vi "example.vi"() -> ()   [LabVIEW 2017, in "libfreenect.lvlib"]
uses:
  libfreenect.lvlib
  <vilib>/Analysis/coordinate.llb/2D Cartesian Coordinate Rotation (Array).vi
  <vilib>/gmath/statdist.llb/Normal PDF.vi
  <vilib>/Analysis/NI_AALPro.lvlib
  <vilib>/gmath/NI_Gmath.lvlib
panel:
  out "KINECT DATA":cluster{dbl[], dbl[]}[](graph)
  in  "Till Angle":dbl(slide) scale=-31.0..31.0 scale format="%#_5g"
  out "Heading":dbl(knob) scale=-180.0..180.0
  in  "Start":bool
  out "Command String":string
  out "Roll":dbl(knob) scale=-180.0..180.0
  out "Pitch":dbl(slide) scale=-90.0..90.0
  in  "Stop Continuous":bool
  out "Error Output":errorcluster
  in  "Serial Port":refnum<visa-resource-name>="COM1"
  in  "Baud Rate":u32=115200
  in  "std":dbl=1.0
  in  "x":dbl=50.0
  in  "y":dbl=50.0
  in  "x":dbl
  in  "y1":dbl
  out "Occupancy Grid Map":dbl[][](graph)
  in  "x1":dbl
  out "z":dbl
  out "y":dbl
  out "x":dbl
  in  "error in (no error)":errorcluster
  out "H-A":dbl
  out "W-A":dbl
  out "Height":dbl
  out "Width":dbl
  out "Depth Image":T1(plugin-control)
  out "RGB Image":T1(plugin-control)
  in  "stop":bool
  out "Range":dbl
  # "KINECT CONTROL BUTTONS"
  # "Pixel Coordinate"
  # "Map Coordinates"
  # "DATA IMAGE"
  # "IMU CONTROL BUTTONS"
  # "IMU DATA"
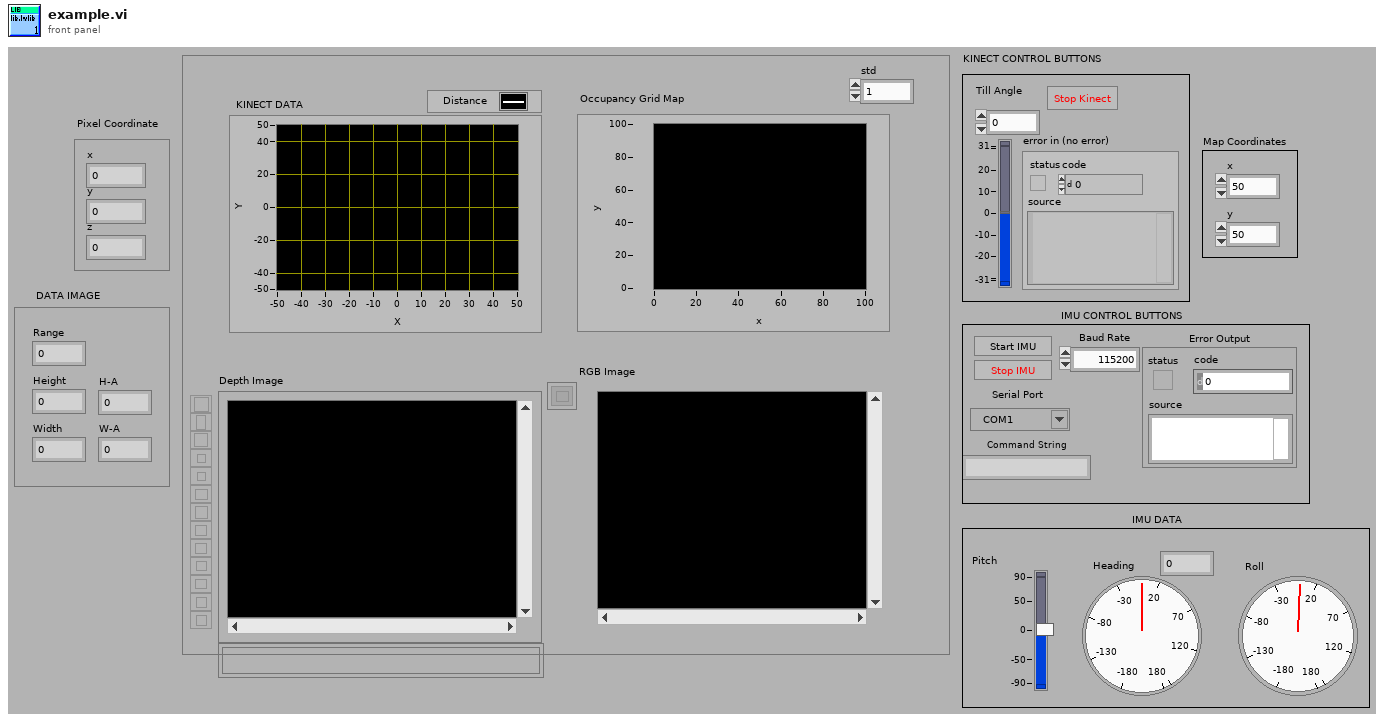
[diagram p1: front panel]
types:
  T1 = typedef "IMAQ Image.ctl" = refnum<image>
  T2 = enum16{"open", "replace", "create", "open or create", "replace or create", "replace or create with confirmation"}
  T3 = typedef "Image Type" = u32
  T4 = enum16{"FREENECT_DEPTH_11BIT", "FREENECT_DEPTH_10BIT", "FREENECT_DEPTH_11BIT_PACKED", "FREENECT_DEPTH_10BIT_PACKED"}
  T5 = enum16{"FREENECT_VIDEO_RGB", "FREENECT_VIDEO_BAYER", "FREENECT_VIDEO_IR_8BIT", "FREENECT_VIDEO_IR_10BIT", "FREENECT_VIDEO_IR_10BIT_PACKED", "FREENECT_VIDEO_YUB_RGB", "FREENECT_VIDEO_YUB_RAW"}
  T6 = cluster{"Cmd/SOP Byte":string, "Header Size":u16, "Len":u16, "Chksum Start":u16, "Chksum End":i16, "InHdr":bool}[]
  T7 = cluster{"Command Byte":u8, "Acceleration Vector":cluster{sgl, sgl, sgl}, "Timer Ticks":u32, "Checksum":u16}
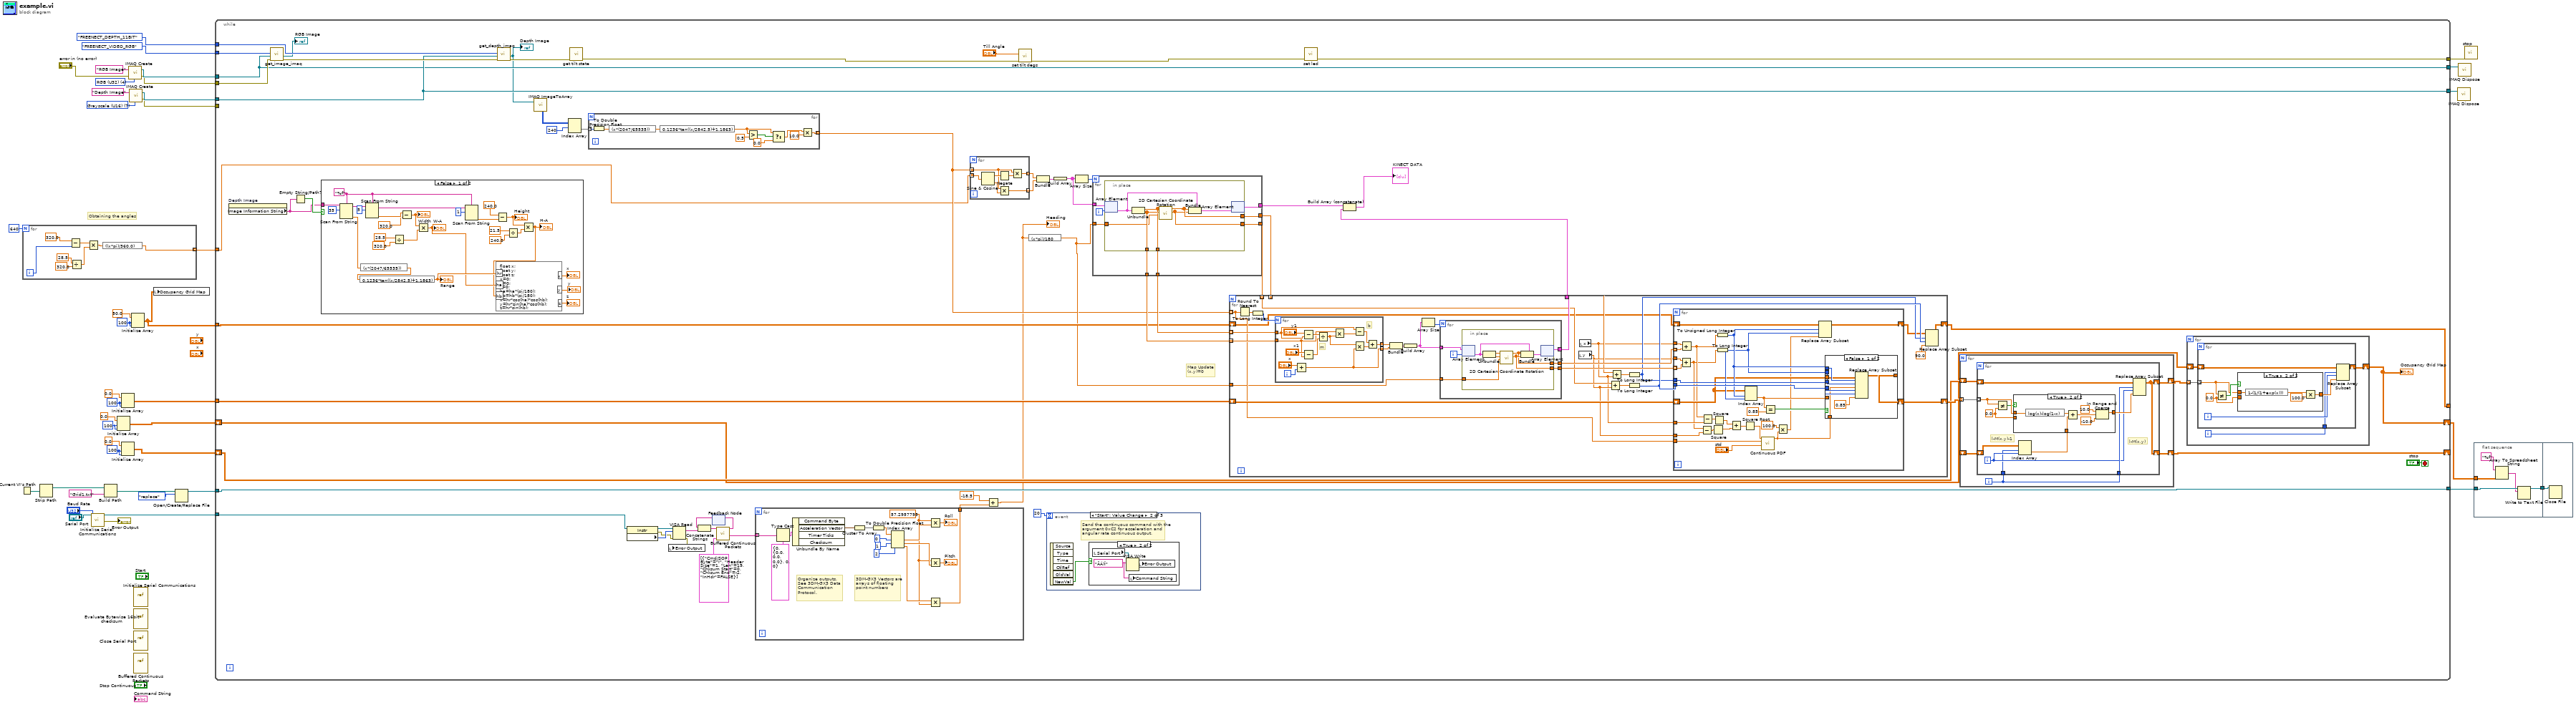
[diagram p0: block diagram]
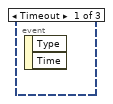
[diagram p2: hidden frame]
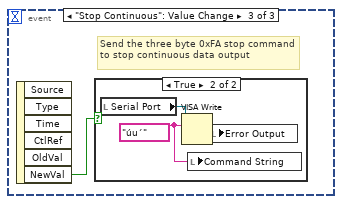
[diagram p4: hidden frame]
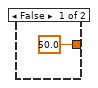
[diagram p6: hidden frame]
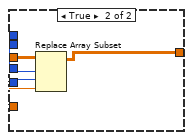
[diagram p8: hidden frame]
diagram:
  w18 = 100 ("dimension size")
  w23 = 100 ("dimension size")
  w24 = 100 ("dimension size")
  w26 = 100 ("dimension size")
  w33 = T3 7 items=["Grayscale (U8)", "Grayscale (I16)", "Grayscale (SGL)", "Complex (CSG)", "RGB (U32)", "HSL (U32)", "RGB (U64)", "Grayscale (U16)"] ("Image Type")
  w38 = T3 4 items=["Grayscale (U8)", "Grayscale (I16)", "Grayscale (SGL)", "Complex (CSG)", "RGB (U32)", "HSL (U32)", "RGB (U64)", "Grayscale (U16)"] ("Image Type")
  # "Obtaining the angles"
  n1 = Current VI's Path() -> (path=w11:path)
  n2 = for {
    N: 640 -> [_]
    tunnel: [w42] -> w2 mode=indexing
    i -> [w43]
    n3 = Subtract(x=320.0, y=w43) -> (x-y=w44:dbl)
    n4 = Divide(x=28.5, y=320.0) -> (x/y=w45:dbl)
    n5 = Multiply(x=w44, y=w45) -> (x*y=w46:dbl)
    n6 = expression code="((x*pi)/360.0)"(w46) -> (w42:dbl)
  }
  n7 = Strip Path(path=w11) -> (stripped path=w14:path)  [unwired: 1 out]
  n8 = call "Initialize Serial Communications.vi"("Serial Port"="Serial Port", "Baud Rate"="Baud Rate") -> ("Serial Port Out"=w4:refnum<visa-resource-name>, "error out"=→"Error Output":errorcluster)  [unwired: 12 in]
  n9 = Build Path(base path=w14, name or relative path="Grid1.txt") -> (appended path=w13:path)
  n10 = Initialize Array(0.0 ("element"), w18, w18) -> (w17:dbl[][])
  n11 = Initialize Array(0.0 ("element"), w24, w24) -> (w20:dbl[][])
  n12 = Initialize Array(0.0 ("element"), w23, w23) -> (w21:dbl[][])
  n13 = call "IMAQ Create"("Image Name"="RGB Image", "Image Type"=w38, "error in (no error)"="error in (no error)") -> ("New Image"=w36:T1, "error out"=w35:errorcluster)  [unwired: 1 in, 1 out]
  n14 = call "IMAQ Create"("Image Name"="Depth Image", "Image Type"=w33) -> ("New Image"=w32:T1, "error out"=w31:errorcluster)  [unwired: 2 in, 1 out]
  n15 = Initialize Array(50.0 ("element"), w26, w26) -> (w16:dbl[][])
  n16 = vi-ref "Initialize Serial Communications.vi"() -> ()  [unwired: 1 out]
  n17 = vi-ref "Evaluate Bytewise 16bit checksum.vi"() -> ()  [unwired: 1 out]
  n18 = vi-ref "Close Serial Port.vi"() -> ()  [unwired: 1 out]
  n19 = vi-ref "Buffered Continuous Packets.vi"() -> ()  [unwired: 1 out]
  n20 = local write "Occupancy Grid Map"(w16) -> ()
  n21 = Open/Create/Replace File(file path (use dialog)=w13, operation (0:open)=T2."replace") -> (refnum out=w10:refnum<file>)  [unwired: 1 in, 5 out]
  n22 = while {
    tunnel: [w50] -> w41
    tunnel: T5."FREENECT_VIDEO_RGB" ("fmt") -> [w106]
    tunnel: T4."FREENECT_DEPTH_11BIT" ("fmt") -> [w102]
    tunnel: w36 -> [w97]
    tunnel: w35 -> [w105]
    tunnel: w32 -> [w99]
    tunnel: w31 -> [_]
    tunnel: [w99] -> w30
    tunnel: [w97] -> w29
    tunnel: w16 -> [w84]
    tunnel: w20 -> [w82]
    shift-right: [w80] -> _
    shift-left: w21 -> [w79]
    shift-right: [w74] -> w1
    shift-left: w17 -> [w77]
    tunnel: w10 -> [w76]
    tunnel: [w76] -> w9
    tunnel: [w75] -> _
    tunnel: w4 -> [w62]
    tunnel: w2 -> [w54]
    stop <- "stop" stop-if-true
    # "Map Update\n(x,y)=0"
    n23 = property on="Depth Image" class="ImageControl"() -> ("Image Information String"=w100:string)  [unwired: 2 in, 2 out]
    n24 = call "get_image_imaq.vi"("error in"=w105, "Image Resource In"=w97, "fmt"=w106) -> ("error out"=w103:errorcluster, "Image Resource Out"=→"RGB Image":T1)  [unwired: 1 in, 6 out]
    n25 = Empty String/Path?(string/path=w100) -> (empty?=w101:bool)
    n26 = case shown="False" w101 {
      tunnel: w100 -> [w330 _]
      frame False {
        w326 = "%f" ("format string")
        n27 = Scan From String(format string=w326, input string=w330, initial scan location=u32 35) -> (remaining string=w329:string, output 1=w323:dbl)  [unwired: 2 in, 2 out]
        n28 = expression code="(x*(2047/65535))"(w323) -> (w324:dbl)
        n29 = expression code="0.1236*tan((x/2842.5)+1.1863)"(w324) -> (w307:dbl)
        "Range" <- w307
        n30 = Scan From String(format string=w326, input string=w329, initial scan location=u32 5) -> (remaining string=w327:string, output 1=w312:dbl)  [unwired: 2 in, 2 out]
        n31 = Divide(x=28.5, y=320.0) -> (x/y=w316:dbl)
        n32 = Subtract(x=w312, y=320.0 ("x")) -> (x-y=w313:dbl)
        "Width" <- w313
        n33 = Multiply(x=w313, y=w316) -> (x*y=w306:dbl)
        "W-A" <- w306
        n34 = Scan From String(format string=w326, input string=w327, initial scan location=u32 1) -> (output 1=w322:dbl)  [unwired: 2 in, 3 out]
        n35 = Subtract(x=240.0, y=w322) -> (x-y=w317:dbl)
        "Height" <- w317
        n36 = Divide(x=21.5, y=240.0) -> (x/y=w318:dbl)
        n37 = Multiply(x=w317, y=w318) -> (x*y=w305:dbl)
        "H-A" <- w305
        n38 = formula code="float x;\nfloat y;\nfloat z;\nx=0;\ny=0;\nz=0;\nha=ha*(pi/180);\nhb=hb*(pi/180);\nx=hr*cos(ha)*cos(hb);\ny=hr*sin(ha)*cos(hb);\nz=hr*sin(hb);"("hr"=w307, "ha"=w306, "hb"=w305) -> ("x"=→"x":dbl, "y"=→"y":dbl, "z"=→"z":dbl)
      }
      frame True {
      }
    }
    n39 = call "get_depth_imaq.vi"("error in"=w103, "Image Resource In"=w99, "fmt"=w102) -> ("error out"=w104:errorcluster, "Image Resource Out"=w96:T1)  [unwired: 1 in, 6 out]
    "Depth Image" <- w96
    n40 = call "IMAQ ImageToArray"("Image"=w96) -> ("Image Pixels (U16)"=w57:u16[][])  [unwired: 3 in, 4 out]
    n41 = Index Array(array=w57, index (row)=240) -> (element=w56:u16[])  [unwired: 1 in]
    n42 = call "get tilt state.vi"("error in (no error)"=w104) -> ("error out"=w83:errorcluster)  [unwired: 1 in, 9 out]
    n43 = for {
      tunnel: w56 -> [w118] mode=indexing
      tunnel: [w114] -> w55 mode=indexing
      n44 = To Double Precision Float(number=w118) -> (double precision float=w117:dbl)
      n45 = expression code="(x*(2047/65535))"(w117) -> (w116:dbl)
      n46 = expression code="0.1236*tan((x/2842.5)+1.1863)"(w116) -> (w110:dbl)
      n47 = Greater?(x=w110, y=0.5) -> (0:w112:bool)
      n48 = Select(t=w110, s=w112, f=0.0) -> (s? t:f=w109:dbl)
      n49 = Multiply(x=w109, y=10.0) -> (x*y=w114:dbl)
    }
    n50 = property class="Instr"(reference=w62) -> (reference out=w66:refnum<visa-resource-name>, error out=w63:errorcluster, "Serial Settings:Number of Bytes at Serial Port"=w65:u32)  [unwired: 1 in]
    n51 = VISA Read(VISA resource name=w66, byte count=w65, error in (no error)=w63) -> (read buffer=w64:string, error out=w68:errorcluster)  [unwired: 2 out]
    n52 = local write "Error Output"(w68) -> ()
    n53 = feedback #1() -> (w67:string)  [unwired: 1 in]
    n54 = Concatenate Strings(w67, w64) -> (w70:string)
    n55 = call "Buffered Continuous Packets.vi"("Input Buffer"=w70, "Packet definitions"=T6 [{"Cmd/SOP Byte"="Î", "Header Size"=1, "Len"=19, "Chksum Start"=0, "Chksum End"=-2, "InHdr"=FALSE}]) -> ("Remainder String"=w71:string, "Valid Records Found"=w72:string[])  [unwired: 4 in, 3 out]
    n56 = feedback-in #1(w71) -> ()
    n57 = for {
      tunnel: w72 -> [w138] mode=indexing
      tunnel: [w127] -> w60
      w130 = 57.2957795 ("x")
      # "3DM-GX3 Vectors are arrays of floating point numbers"
      # "Organize outputs.  See 3DM-GX3 Data Communication Protocol."
      n58 = Type Cast(type=T7 {"Command Byte"=0, "Acceleration Vector"={0.0, 0.0, 0.0}, "Timer Ticks"=0, "Checksum"=0}, x=w138) -> (*(type *) &x=w141:T7)
      n59 = Unbundle By Name(w141) -> ("Acceleration Vector"=w140:cluster{sgl, sgl, sgl})  [unwired: 3 out]
      n60 = Cluster To Array(cluster=w140) -> (array=w139:sgl[])
      n61 = To Double Precision Float(number=w139) -> (double precision float=w137:dbl[])
      n62 = Index Array(array=w137, index #1=0 ("index"), index #2=1 ("index"), index #3=2 ("index")) -> (element #1=w133:dbl, element #2=w132:dbl, element #3=w131:dbl)
      n63 = Multiply(x=w130, y=w133) -> (x*y=→"Roll":dbl)
      n64 = Multiply(x=w130, y=w132) -> (x*y=→"Pitch":dbl)
      n65 = Multiply(x=w131, y=w130) -> (x*y=w127:dbl)
    }
    n66 = for {
      tunnel: w55 -> [w298] mode=indexing
      tunnel: w54 -> [w299] mode=indexing
      tunnel: [w302] -> w94 mode=indexing
      tunnel: [w301] -> w95 mode=indexing
      n67 = Sine & Cosine(0:w299) -> (1:w304:dbl, 2:w303:dbl)
      n68 = Negate(x=w304) -> (-x=w300:dbl)
      n69 = Multiply(x=w298, y=w303) -> (x*y=w301:dbl)
      n70 = Multiply(x=w298, y=w300) -> (x*y=w302:dbl)
    }
    n71 = Add(x=-18.5, y=w60) -> (x+y=w52:dbl)
    "Heading" <- w52
    n72 = call "set tilt degs.vi"("error in (no error)"=w83, "angle"="Till Angle") -> ("error out"=w107:errorcluster)  [unwired: 1 in, 8 out]
    n73 = expression code="(x*pi)/180"(w52) -> (w61:dbl)
    n74 = Bundle(w94, w95) -> (w89:cluster{dbl[], dbl[]})  [unwired: 1 out]
    n75 = event shown="[1] \"Start\": Value Change" {
      selector: _ -> [_ _ _]
      dyn-events: _ -> [_ _ _]
      timeout: 20 -> [_ _ _]
      event Timeout {
        n76 = event-data() -> ()  [unwired: 1 in, 2 out]
      }
      event "Start": Value Change {
        # "Send the continuous command with the argument 0xC2 for acceleration and angular rate continuous output."
        n77 = event-data() -> ("NewVal"=w119:bool)  [unwired: 1 in, 5 out]
        n78 = case shown="True" w119 {
          frame False {
          }
          frame True {
            w120 = "ÄÁ)Î" ("write buffer")
            n79 = local read "Serial Port"() -> (w122:refnum<visa-resource-name>)
            n80 = VISA Write(VISA resource name=w122, write buffer=w120) -> (error out=w121:errorcluster)  [unwired: 1 in, 2 out]
            n81 = local write "Command String"(w120) -> ()
            n82 = local write "Error Output"(w121) -> ()
          }
        }
      }
      event "Stop Continuous": Value Change {
        # "Send the three byte 0xFA stop command to stop continuous data output"
        n83 = event-data() -> ("NewVal"=w123:bool)  [unwired: 1 in, 5 out]
        n84 = case shown="True" w123 {
          frame False {
          }
          frame True {
            w124 = "úu´" ("write buffer")
            n85 = local read "Serial Port"() -> (w126:refnum<visa-resource-name>)
            n86 = VISA Write(VISA resource name=w126, write buffer=w124) -> (error out=w125:errorcluster)  [unwired: 1 in, 2 out]
            n87 = local write "Command String"(w124) -> ()
            n88 = local write "Error Output"(w125) -> ()
          }
        }
      }
    }
    n89 = Build Array(w89) -> (w92:cluster{dbl[], dbl[]}[])
    n90 = Array Size(array=w92) -> (size(s)=w93:i32)
    n91 = for {
      N: w93 -> [_]
      tunnel: w92 -> [w290]
      tunnel: [w286] -> w88
      tunnel: [w288] -> w91
      tunnel: [w287] -> w90
      tunnel: w61 -> [w285]
      tunnel: [w284] -> w86
      tunnel: [w283] -> w85
      i -> [w289]
      n92 = in-place {
        in-place-border: [w294] -> w288
        in-place-border: [w295] -> w287
        in-place-border: w285 -> [w293]
        in-place-border: [w292] -> w284
        in-place-border: [w291] -> w283
        n93 = in-place-array #2(w290, w289) -> (w297:cluster{dbl[], dbl[]})
        n94 = Unbundle(w297) -> (w294:dbl[], w295:dbl[])
        n95 = call-poly <vilib>:"2D Cartesian Coordinate Rotation.vi"("theta"=w293, "Y"=w295, "X"=w294) -> ("Y Out"=w291:dbl[], "X Out"=w292:dbl[])  [unwired: 6 in, 1 out]
        n96 = Bundle(cluster=w297, w292, w291) -> (w296:cluster{dbl[], dbl[]})
        n97 = in-place-array #2(w296) -> (w286:cluster{dbl[], dbl[]}[])  [unwired: 1 out]
      }
    }
    n98 = for {
      tunnel: w91 -> [w200] mode=indexing
      tunnel: w90 -> [w199] mode=indexing
      tunnel: w55 -> [w192] mode=indexing
      tunnel: [w201] -> w87
      tunnel: w86 -> [w191] mode=indexing
      tunnel: w85 -> [w194] mode=indexing
      shift-right: [w186] -> w75
      shift-left: w84 -> [w188]
      shift-right: [w193] -> w81
      shift-left: w82 -> [w196]
      tunnel: w61 -> [w185]
      n99 = Round To Nearest(number=w192) -> (nearest integer value=w202:dbl)
      n100 = To Long Integer(number=w202) -> (32bit integer=w195:i32)
      n101 = for {
        N: w195 -> [_]
        tunnel: [w275] -> w204 mode=indexing
        tunnel: [w271] -> w205 mode=indexing
        tunnel: w199 -> [w273]
        tunnel: w200 -> [w274]
        i -> [w270]
        # "m"
        # "b"
        n102 = Add(x="x", y=w270) -> (x+y=w271:dbl)
        n103 = Subtract(x="y1", y=w274) -> (x-y=w280:dbl)
        n104 = Subtract(x="x1", y=w273) -> (x-y=w279:dbl)
        n105 = Divide(x=w280, y=w279) -> (x/y=w277:dbl)
        n106 = Multiply(x=w273, y=w277) -> (x*y=w278:dbl)
        n107 = Subtract(x=w274, y=w278) -> (x-y=w276:dbl)
        n108 = Multiply(x=w277, y=w271) -> (x*y=w272:dbl)
        n109 = Add(x=w276, y=w272) -> (x+y=w275:dbl)
      }
      n110 = Bundle(w204, w205) -> (w210:cluster{dbl[], dbl[]})  [unwired: 1 out]
      n111 = Build Array(w210) -> (w211:cluster{dbl[], dbl[]}[])
      n112 = Array Size(array=w211) -> (size(s)=w212:i32)
      n113 = for {
        N: w212 -> [_]
        tunnel: w211 -> [w261]
        tunnel: [w259] -> w201
        tunnel: [w258] -> w208
        tunnel: [w257] -> w209
        tunnel: w185 -> [w256]
        i -> [w260]
        n114 = in-place {
          in-place-border: [w264] -> w258
          in-place-border: [w263] -> w257
          in-place-border: w256 -> [w262]
          n115 = in-place-array #3(w261, w260) -> (w266:cluster{dbl[], dbl[]})
          n116 = Unbundle(w266) -> (w268:dbl[], w267:dbl[])
          n117 = call-poly <vilib>:"2D Cartesian Coordinate Rotation.vi"("theta"=w262, "Y"=w267, "X"=w268) -> ("Y Out"=w264:dbl[], "X Out"=w263:dbl[])  [unwired: 6 in, 1 out]
          n118 = Bundle(cluster=w266, w263, w264) -> (w265:cluster{dbl[], dbl[]})
          n119 = in-place-array #3(w265) -> (w259:cluster{dbl[], dbl[]}[])  [unwired: 1 out]
        }
      }
      n120 = local read "y"() -> (w190:dbl)
      n121 = local read "x"() -> (w189:dbl)
      n122 = Add(x=w194, y=w190) -> (x+y=w207:dbl)
      n123 = Add(x=w191, y=w189) -> (x+y=w206:dbl)
      n124 = To Long Integer(number=w206) -> (32bit integer=w197:i32)
      n125 = To Long Integer(number=w207) -> (32bit integer=w198:i32)
      n126 = for {
        tunnel: w209 -> [w225] mode=indexing
        tunnel: w208 -> [w224] mode=indexing
        tunnel: w189 -> [w227]
        tunnel: w190 -> [w226]
        shift-right: [w216] -> w187
        shift-left: w188 -> [w217]
        tunnel: w197 -> [w242]
        tunnel: w198 -> [w241]
        shift-right: [w237] -> w193
        shift-left: w196 -> [w238]
        tunnel: w189 -> [w221]
        tunnel: w190 -> [w219]
        tunnel: w192 -> [w218]
        n127 = Add(x=w226, y=w224) -> (x+y=w220:dbl)
        n128 = Add(x=w227, y=w225) -> (x+y=w222:dbl)
        n129 = Subtract(x=w220, y=w219) -> (x-y=w228:dbl)
        n130 = Subtract(x=w222, y=w221) -> (x-y=w229:dbl)
        n131 = Square(x=w228) -> (x^2=w230:dbl)
        n132 = Square(x=w229) -> (x^2=w231:dbl)
        n133 = To Unsigned Long Integer(number=w222) -> (unsigned 32bit integer=w240:u32)
        n134 = To Long Integer(number=w220) -> (32bit integer=w239:i32)
        n135 = Add(x=w231, y=w230) -> (x+y=w232:dbl)
        n136 = Square Root(x=w232) -> (sqrt(x)=w233:dbl)
        n137 = Index Array(array=w238, index (row)=w240, index (col)=w239) -> (element=w235:dbl)
        n138 = call-poly <vilib>:"Continuous PDF.vi"("std"="std", "mean"=w218, "x"=w233) -> ("pdf(x)"=w215:dbl)  [unwired: 7 in, 1 out]
        n139 = Equal?(x=w235, y=0.85 ("x")) -> (x = y?=w236:bool)
        n140 = Multiply(x=100.0, y=w215) -> (x*y=w213:dbl)
        n141 = Replace Array Subset(array=w217, new element=w213, index (row)=w240, index (col)=w239) -> (w216:dbl[][])
        n142 = case shown="False" w236 {
          tunnel: w242 -> [w249 _]
          tunnel: w241 -> [w248 _]
          tunnel: w240 -> [w247 w252]
          tunnel: w239 -> [w246 w253]
          tunnel: w238 -> [w245 w255]
          tunnel: [w244 w251] -> w237
          tunnel: w235 -> [_ w254]
          tunnel: w215 -> [w243 _]
          frame False {
            n143 = Replace Array Subset(array=w245, new element #1=w243, index (row) #1=w247, index (col) #1=w246, new element #2=0.85 ("new element/subarray"), index (row) #2=w249, index (col) #2=w248) -> (w244:dbl[][])
          }
          frame True {
            n144 = Replace Array Subset(array=w255, new element=w254, index (row)=w252, index (col)=w253) -> (w251:dbl[][])
          }
        }
      }
      n145 = Replace Array Subset(array=w187, new element=90.0 ("new element/subarray"), index (row)=w197, index (col)=w198) -> (w186:dbl[][])
    }
    n146 = call "set led.vi"("error in (no error)"=w107) -> ("error out"=w50:errorcluster)  [unwired: 2 in, 8 out]
    n147 = Build Array (concatenate)(w88, w87) -> (→"KINECT DATA":cluster{dbl[], dbl[]}[])
    n148 = for {
      tunnel: w81 -> [w165] mode=indexing
      shift-right: [w163] -> w80
      shift-left: _ -> [w164]
      shift-right: [w160] -> w78
      shift-left: w79 -> [w161]
      i -> [w162]
      n149 = for {
        tunnel: w165 -> [w176] mode=indexing
        shift-right: [w166] -> w163
        shift-left: w164 -> [w170]
        tunnel: w162 -> [w174]
        tunnel: w162 -> [w172]
        shift-right: [w166] -> w160
        shift-left: w161 -> [w167]
        i -> [w173]
        w168 = 0.0 ("y")
        # "l-M(x,y)-1"
        # "l-M(x,y)"
        n150 = Not Equal?(x=w176, y=w168) -> (x != y?=w169:bool)
        n151 = Index Array(array=w170, index (row)=w172, index (col)=w173) -> (element=w171:dbl)
        n152 = case shown="True" w169 {
          tunnel: w176 -> [_ w184]
          tunnel: [w177 w180] -> w175
          tunnel: w171 -> [w177 w183]
          tunnel: w168 -> [_ _]
          frame False {
          }
          frame True {
            n153 = expression code="log(x)-log(1-x)"(w184) -> (w182:dbl)
            n154 = Add(x=w182, y=w183) -> (x+y=w181:dbl)
            n155 = In Range and Coerce(upper limit=10.0, x=w181, lower limit=-10.0) -> (coerced(x)=w180:dbl)  [unwired: 1 out]
          }
        }
        n156 = Replace Array Subset(array=w167, new element=w175, index (row)=w174, index (col)=w173) -> (w166:dbl[][])
      }
    }
    n157 = for {
      tunnel: w78 -> [w146] mode=indexing
      shift-right: [w144] -> w74
      shift-left: w77 -> [w145]
      i -> [w143]
      n158 = for {
        tunnel: w146 -> [w153] mode=indexing
        tunnel: w143 -> [w147]
        shift-right: [w151] -> w144
        shift-left: w145 -> [w152]
        i -> [w148]
        w149 = 0.0 ("y")
        n159 = Not Equal?(x=w153, y=w149) -> (x != y?=w154:bool)
        n160 = case shown="True" w154 {
          tunnel: w153 -> [_ w159]
          tunnel: [50.0 w156] -> w150
          tunnel: w149 -> [_ _]
          frame False {
          }
          frame True {
            n161 = expression code="1-(1/(1+exp(x)))"(w159) -> (w158:dbl)
            n162 = Multiply(x=w158, y=100.0) -> (x*y=w156:dbl)
          }
        }
        n163 = Replace Array Subset(array=w152, new element=w150, index (row)=w147, index (col)=w148) -> (w151:dbl[][])
      }
    }
    "Occupancy Grid Map" <- w74
  }
  n164 = call "IMAQ Dispose"("Image"=w30) -> ()  [unwired: 2 in, 4 out]
  n165 = call "IMAQ Dispose"("Image"=w29) -> ()  [unwired: 2 in, 4 out]
  n166 = call "stop.vi"("error in (no error)"=w41) -> ()  [unwired: 11 out]
  n167 = flat-sequence {
    tunnel: w1 -> [w336]
    tunnel: w9 -> [w334]
    tunnel: [w332] -> w8
    tunnel: w8 -> [w337]
    frame #0 {
      n168 = Array To Spreadsheet String(array=w336, 3:"%f" ("format string")) -> (spreadsheet string=w333:string)  [unwired: 1 in]
      n169 = Write to Text File(file (use dialog)=w334, text=w333) -> (refnum out=w332:refnum<file>)  [unwired: 1 in, 3 out]
    }
    frame #1 {
      n170 = Close File(refnum=w337) -> ()  [unwired: 1 in, 2 out]
    }
  }
